vi "Wait For Acquisition By Handle Time Out.vi"(10 "iTimeOutMs":i32, 11 "cameraHandle":i32) -> (3 "function return":u32)   [LabVIEW 2018, in "AndorSDK.lvlib"]
doc: "EXPNETTYPE unsigned int WINAPI WaitForAcquisitionByHandleTimeOut(long cameraHandle, int iTimeOutMs);"
uses:
  AndorSDK.lvlib
  ATMCD32D.dll
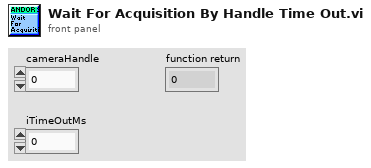
[diagram p1: front panel]
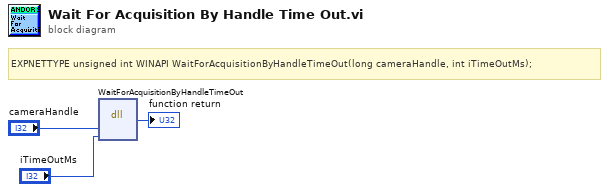
[diagram p0: block diagram]
diagram:
  # "EXPNETTYPE unsigned int WINAPI WaitForAcquisitionByHandleTimeOut(long cameraHandle, int iTimeOutMs);"
  n1 = dll-call lib="PTH2babs E\nPersönliches02 - Arbeit03-HiwijobsLabviewCodelibANDOR\tAndor SDK\nATMCD32D.*" fn="WaitForAcquisitionByHandleTimeOut"("cameraHandle"="cameraHandle", "iTimeOutMs"="iTimeOutMs") -> (→"function return":u32)  [unwired: 5 in, 2 out]
